vi "Finish Command.vi"(8 "error in":errorcluster) -> (0 "error out":errorcluster)   [LabVIEW 2016, in "Drive System.lvlib"]
uses:
  Drive System.lvlib
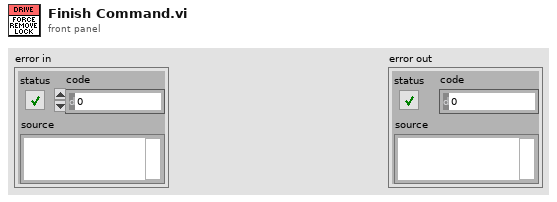
[diagram p1: front panel]
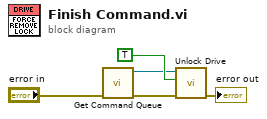
[diagram p0: block diagram]
diagram:
  n1 = call "Get Command Queue.vi"("error in (no error)"="error in") -> ("error out"=w2:errorcluster, "Queue out"=w4:refnum<queue>)  [unwired: 9 in]
  n2 = call "Unlock Drive.vi"("error in"=w2, "Force"=TRUE, "Queue in"=w4) -> ("error out"=→"error out":errorcluster)  [unwired: 8 in]
